vi "Configure Line Sync.vi"(8 "error in (no error)":errorcluster, 11 "VISA resource name":refnum<visa-resource-name>) -> (0 "error out":errorcluster, 3 "VISA resource name out":refnum<visa-resource-name>)   [LabVIEW 2018, in "Keithley DMM7512.lvlib"]
doc: "This VI configures if line synchronization is used during the measurement."
uses:
  <instrlib>/Keithley DMM7512/Keithley DMM7512.lvlib
panel:
  in  "Function":u16(ring) items=["Voltage: DC", "Voltage: AC", "Current: DC", "Current: AC", "2W Resistance", "4W Resistance", "Diode", "Capacitance", "Temperature", "Continuity", "Frequency", "Period", "Ratio", "Digitize Voltage", "Digitize Current"]
  in  "State":bool
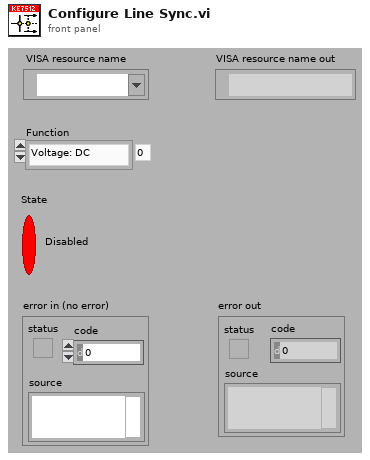
[diagram p1: front panel]
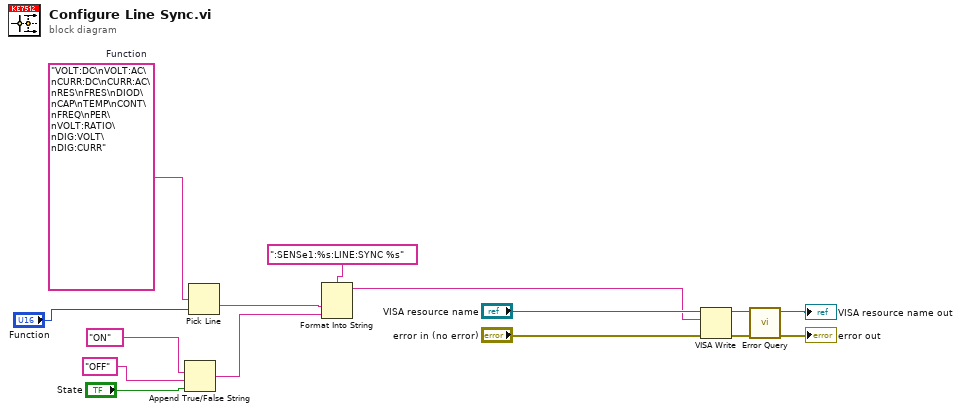
[diagram p0: block diagram]
diagram:
  w2 = "VOLT:DC\nVOLT:AC\nCURR:DC\nCURR:AC\nRES\nFRES\nDIOD\nCAP\nTEMP\nCONT\nFREQ\nPER\nVOLT:RATIO\nDIG:VOLT\nDIG:CURR"  # Function
  n1 = Append True/False String(1:"State", 2:"OFF", 3:"ON") -> (0:w3:string)  [unwired: 1 in]
  n2 = Pick Line(multi-line string=w2, line index="Function") -> (output string=w8:string)  [unwired: 1 out]
  n3 = Format Into String(format string=":SENSe1:%s:LINE:SYNC %s", w8, w3) -> (resulting string=w7:string)  [unwired: 2 in, 1 out]
  n4 = VISA Write(VISA resource name="VISA resource name", write buffer=w7, error in (no error)="error in (no error)") -> (VISA resource name out=w13:refnum<visa-resource-name>, error out=w10:errorcluster)  [unwired: 1 out]
  n5 = call <instrlib>:"Error Query.vi"("error in (no error)"=w10, "VISA resource name"=w13) -> ("error out"=→"error out":errorcluster, "VISA resource name out"=→"VISA resource name out":refnum<visa-resource-name>)  [unwired: 8 out]
